vi "TIFF Add Img IFD.vi"   [LabVIEW 2016]
uses:
  Class/TIFF/TIFF.lvclass
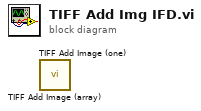
[diagram p0: block diagram]
diagram:
  n1 = call-dynamic "TIFF Add Image (array).vi"() -> ()  [unwired: 10 in, 2 out]
  n2 = call-dynamic "TIFF Add Image (one).vi"() -> ()  [unwired: 10 in, 2 out]
